vi "flattern_to_json.vi"() -> ()   [LabVIEW 2022 SP3]
panel:
  out "value":cluster{"data":dbl, "string":string[]}
  out "JSON string":string
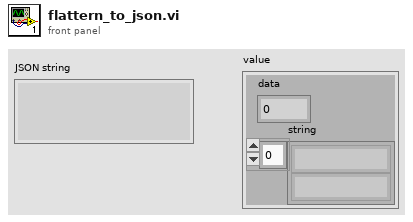
[diagram p1: front panel]
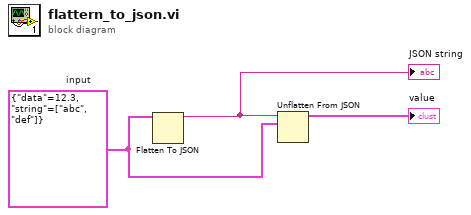
[diagram p0: block diagram]
diagram:
  w2 = cluster{"data":dbl, "string":string[]} {"data"=12.3, "string"=["abc", "def"]}  # input
  n1 = Flatten To JSON(anything=w2) -> (JSON string=w3:string)  [unwired: 2 in, 1 out]
  "JSON string" <- w3
  n2 = Unflatten From JSON(JSON string=w3, type and defaults=w2) -> (value=→"value":cluster{"data":dbl, "string":string[]})  [unwired: 5 in, 1 out]
